vi "Output_file_Panel.vi"(8 "Show panel ?":bool, 9 "Channel Names":string[](array[string]), 10 "Header":string, 11 "Output filename":path=path "/G3_3 HD/Users/Paul/New Disp DB file") -> (0 "Save Full Res Data?":bool, 1 "Desired Columns":i32[](array[numeric]), 2 "Header Out":string, 3 "Output filename Out":path=path "/G3_3 HD/Users/Paul/New Disp DB file", 4 "Channels to Tabulate in header Out":i32[](listbox), 5 "Save Plotted rows only?":bool, 6 "Summarise mode":T1(ring), 7 "Grouping info":T3[](array[typedef]))   [LabVIEW 2016]
uses:
  Controls/Group_Binning.ctl
  Results_plotter_Global.vi
panel:
  out "Raw data file index":i32
  in  "Channels to Tabulate in header":i32[](listbox)
  in  "Channels to first \"bin\" then output":i32[](listbox)
  in  "Channels to Ouput":i32[](listbox)
  in  "Channel to bin":T2(array[cluster])
  in  "Summarize data":i32(listbox)=2
  in  "OK Button":bool
  in  "Column Selector":i32(listbox)
  in  "Row Selector":i32(listbox)=1
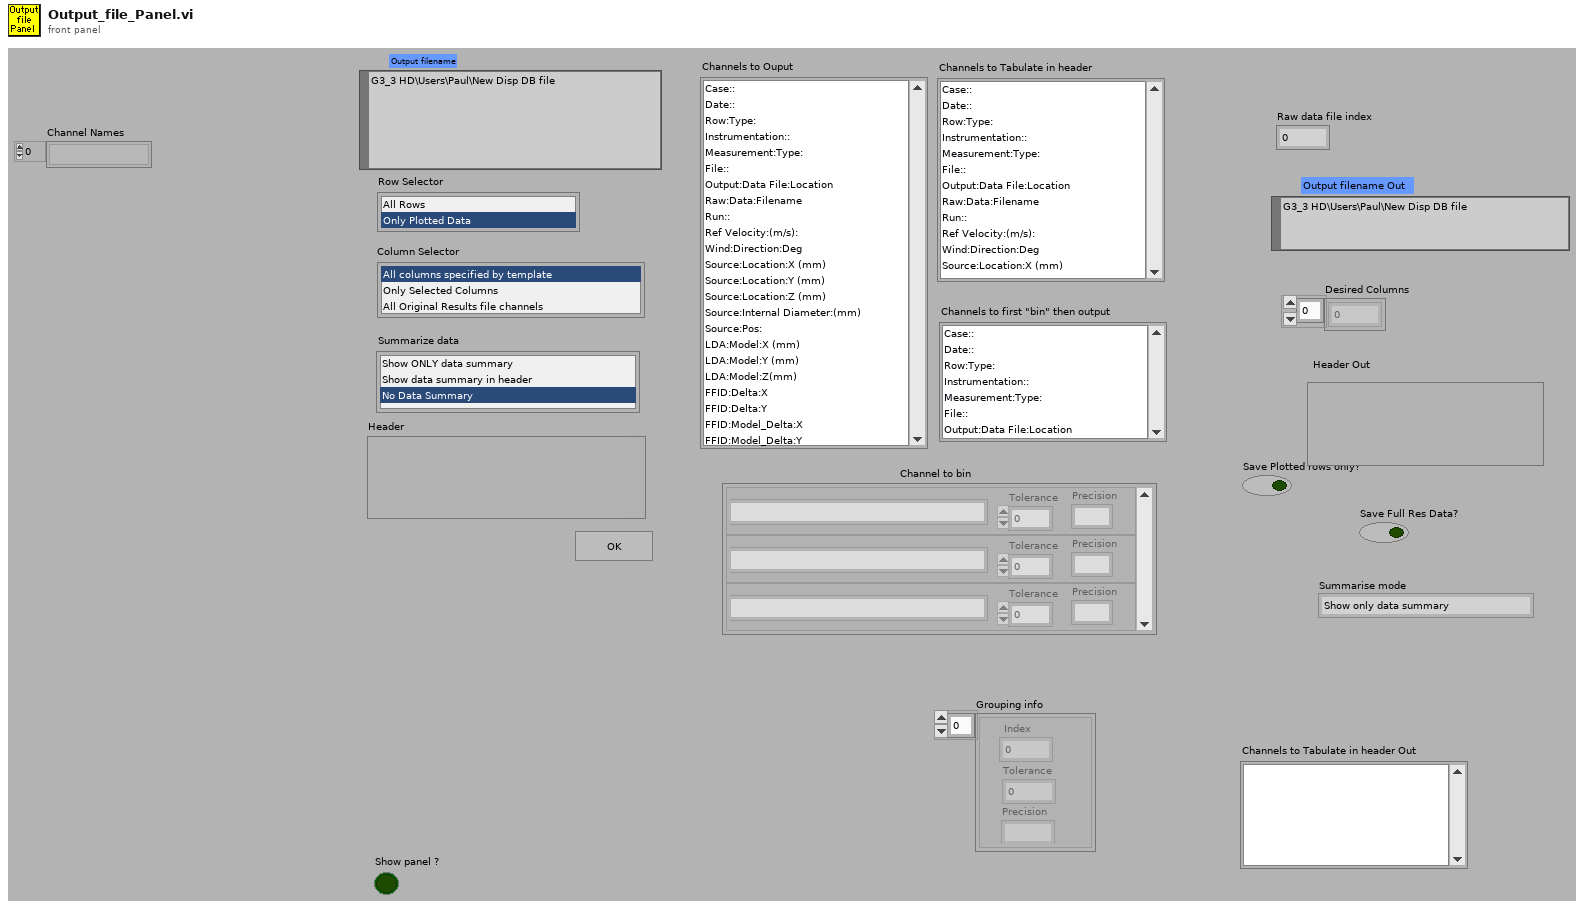
[diagram p1: front panel]
types:
  T1 = enum16{"Show only data summary", "Show data summary", "No data summary"}
  T2 = cluster{"Ch Name":string, "Tolerance":dbl, "Precision":string}[]
  T3 = typedef "Group_Binning.ctl" = cluster{"Index":i32, "Tolerance":dbl, "Precision":string}
  T4 = typedef "Dispose_Channel.ctl" = enum16{"Always", "If Blank", "Never"}
  T5 = cluster{"Ch Name":string, "Tolerance":dbl, "Precision":string}
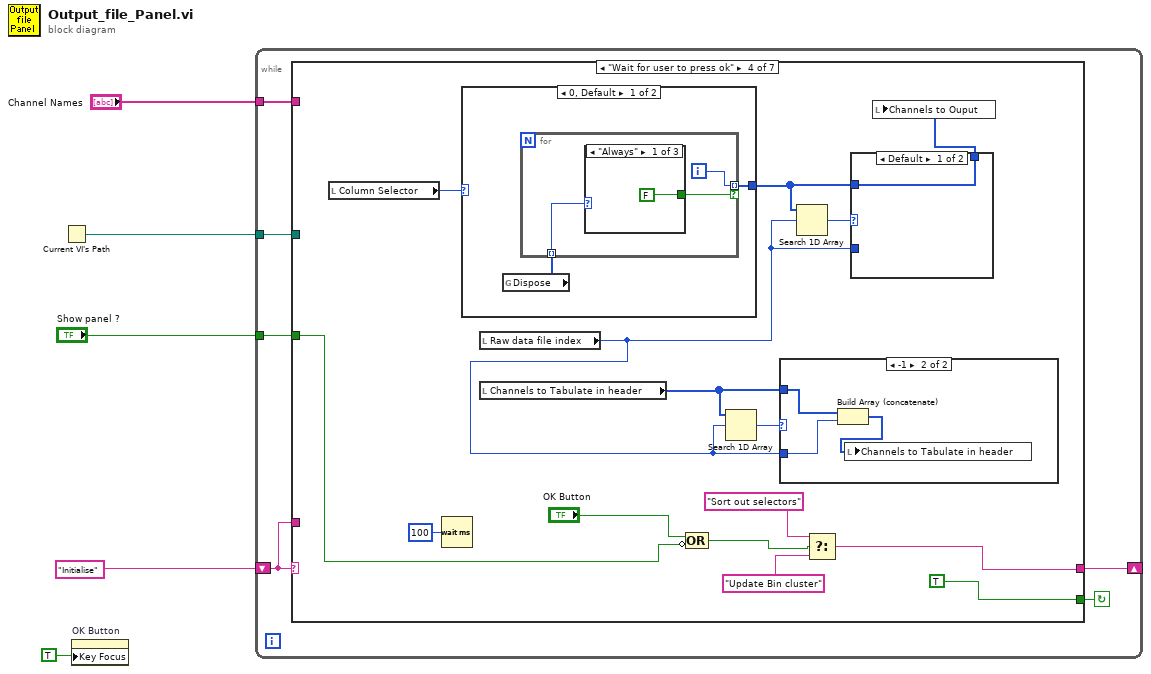
[diagram p0: block diagram]
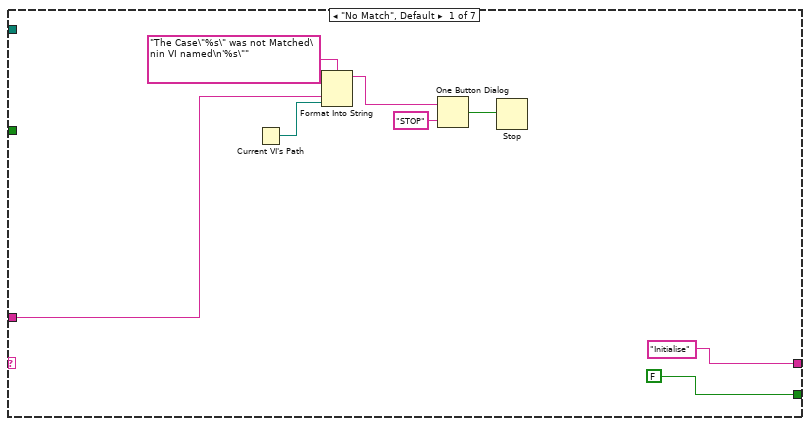
[diagram p2: hidden frame]
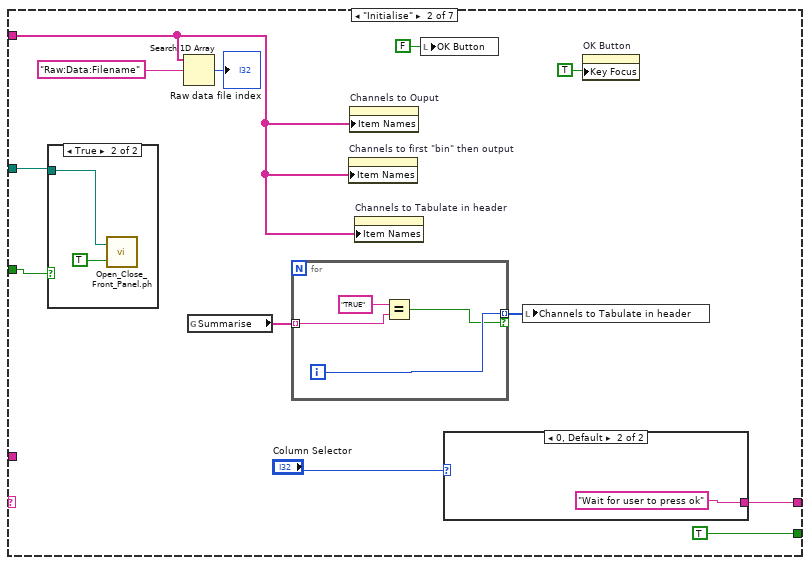
[diagram p3: hidden frame]
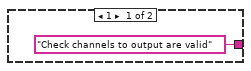
[diagram p4: hidden frame]
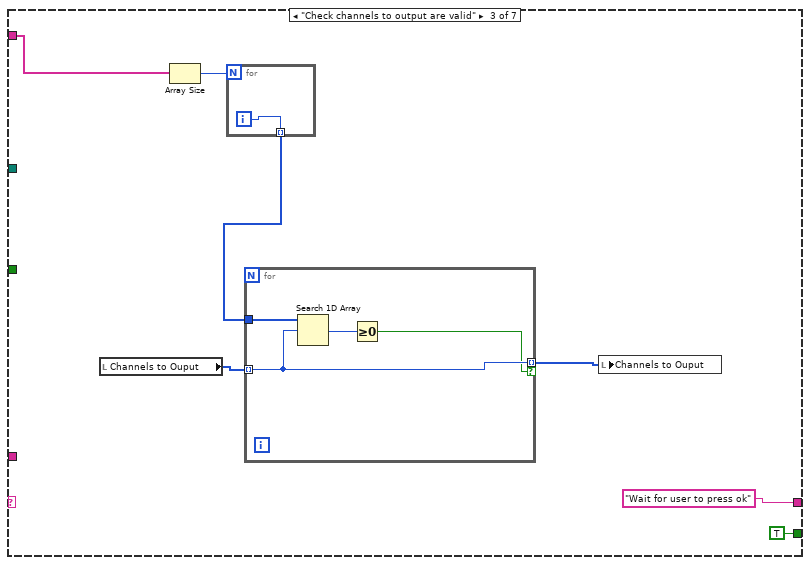
[diagram p6: hidden frame]
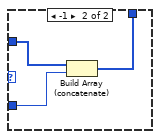
[diagram p8: hidden frame]
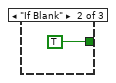
[diagram p9: hidden frame]
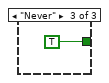
[diagram p10: hidden frame]
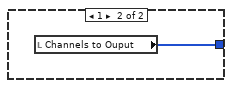
[diagram p11: hidden frame]
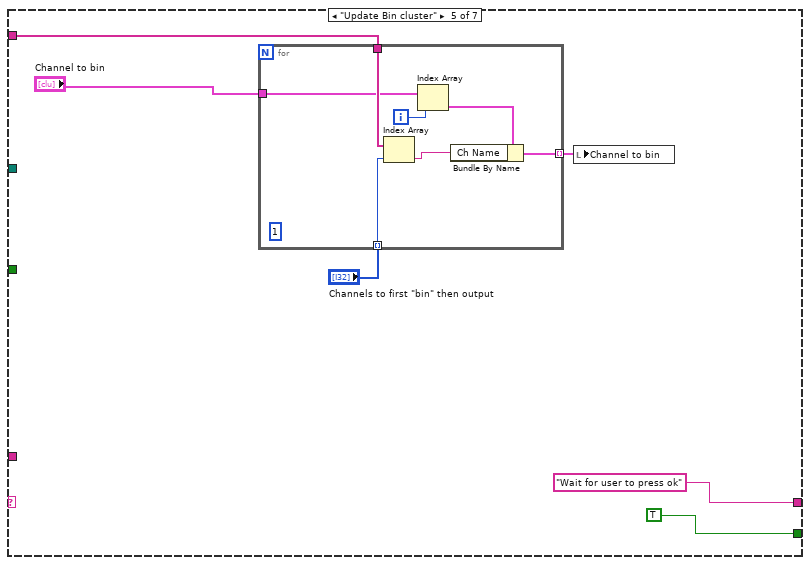
[diagram p12: hidden frame]
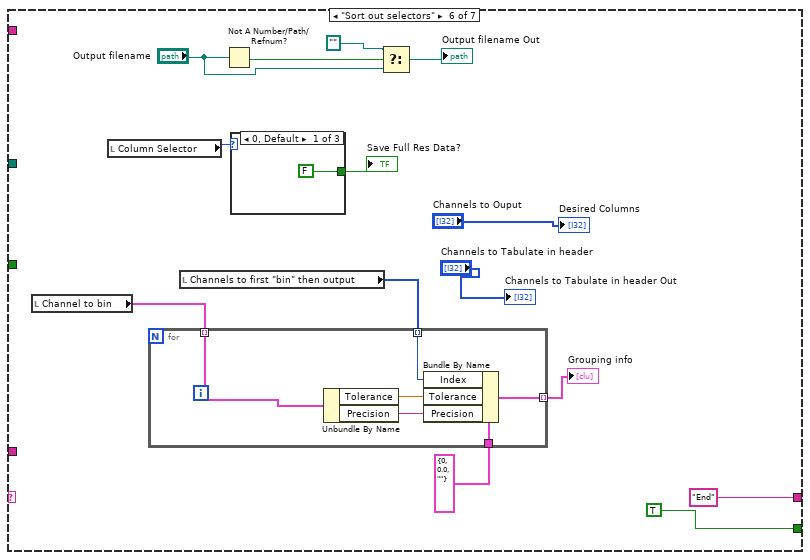
[diagram p13: hidden frame]
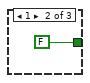
[diagram p14: hidden frame]
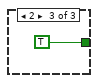
[diagram p15: hidden frame]
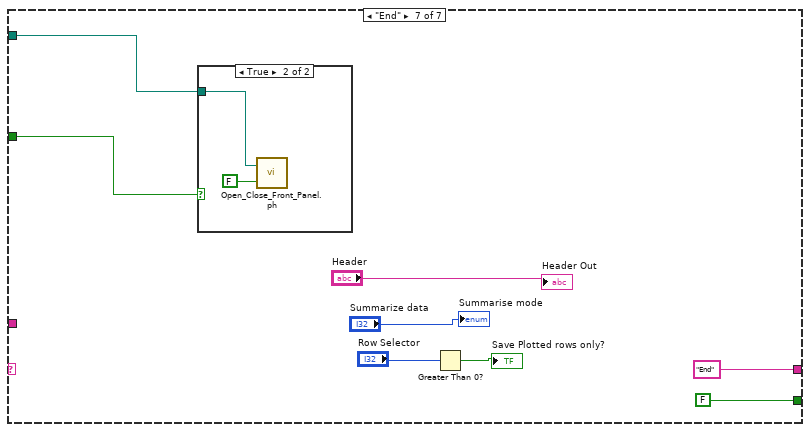
[diagram p16: hidden frame]
diagram:
  n1 = Current VI's Path() -> (path=w3:path)
  n2 = property on="OK Button" class="Bool (strict)"("Key Focus"=TRUE) -> ()  [unwired: 2 in, 2 out]
  n3 = while {
    shift-left: "Initialise" -> [w9]
    shift-right: [w10] -> _
    tunnel: "Show panel ?" -> [w8]
    tunnel: w3 -> [w7]
    tunnel: "Channel Names" -> [w6]
    stop <- w11 continue-if-true
    n4 = case shown="\"Wait for user to press ok\"" w9 {
      tunnel: [FALSE TRUE TRUE TRUE TRUE TRUE FALSE] -> w11
      tunnel: ["Initialise" w31 "Wait for user to press ok" w65 "Wait for user to press ok" "End" ("t") "End"] -> w10
      tunnel: w9 -> [w14 _ _ _ _ _ _]
      tunnel: w8 -> [_ w28 _ w59 _ _ w124]
      tunnel: w7 -> [_ w29 _ _ _ _ w123]
      tunnel: w6 -> [_ w21 w45 _ w85 _ _]
      frame "No Match", Default {
        n5 = Current VI's Path() -> (path=w13:path)
        n6 = Format Into String(format string="The Case\"%s\" was not Matched\nin VI named\n'%s\"" ("Format String"), w14, w13) -> (resulting string=w17:string)  [unwired: 2 in, 1 out]
        n7 = One Button Dialog(message=w17, button name ("OK")="STOP") -> (true=w15:bool)
        n8 = Stop(stop? (T)=w15) -> ()
      }
      frame "Initialise" {
        n9 = case shown="True" w28 {
          tunnel: w29 -> [_ w35]
          frame False {
          }
          frame True {
            n10 = call "Open_Close_Front_Panel.ph.vi"("Front Panel Window:Open"=TRUE, "VI path"=w35) -> ()  [unwired: 2 out]
          }
        }
        n11 = Search 1D Array(1D array=w21, element="Raw:Data:Filename" ("y")) -> (index of element=→"Raw data file index":i32)  [unwired: 1 in]
        n12 = global read "Results_plotter_Global.vi" "Summarise"() -> (w25:string[])
        n13 = for {
          tunnel: w25 -> [w38] mode=indexing
          tunnel: [w37] -> w24 mode=indexing if=w36
          i -> [w37]
          n14 = Equal?(x="TRUE", y=w38) -> (x = y?=w36:bool)
        }
        n15 = property on="Channels to first \"bin\" then output" class="LstBox (strict)"("Item Names"=w21) -> ()  [unwired: 2 in, 2 out]
        n16 = property on="Channels to Ouput" class="LstBox (strict)"("Item Names"=w21) -> ()  [unwired: 2 in, 2 out]
        n17 = property on="Channels to Tabulate in header" class="LstBox (strict)"("Item Names"=w21) -> ()  [unwired: 2 in, 2 out]
        n18 = local write "OK Button"(FALSE ("OK Button")) -> ()
        n19 = case shown="0, Default" "Column Selector" {
          tunnel: ["Check channels to output are valid" "Wait for user to press ok"] -> w31
          frame 1 {
          }
          frame 0, Default {
          }
        }
        n20 = local write "Channels to Tabulate in header"(w24) -> ()
        n21 = property on="OK Button" class="Bool (strict)"("Key Focus"=TRUE) -> ()  [unwired: 2 in, 2 out]
      }
      frame "Check channels to output are valid" {
        n22 = local read "Channels to Ouput"() -> (w44:i32[])
        n23 = Array Size(array=w45) -> (size(s)=w46:i32)
        n24 = for {
          N: w46 -> [_]
          tunnel: [w51] -> w43 mode=indexing
          i -> [w51]
        }
        n25 = for {
          tunnel: w44 -> [w49] mode=indexing
          tunnel: w43 -> [w50]
          tunnel: [w49] -> w42 mode=indexing if=w47
          n26 = Search 1D Array(1D array=w50, element=w49) -> (index of element=w48:i32)  [unwired: 1 in]
          n27 = Greater Or Equal To 0?(x=w48) -> (x >= 0?=w47:bool)
        }
        n28 = local write "Channels to Ouput"(w42) -> ()
      }
      frame "Wait for user to press ok" {
        n29 = local read "Column Selector"() -> (w52:i32)
        n30 = Wait (ms)(milliseconds to wait=u32 100) -> ()  [unwired: 1 out]
        n31 = case shown="0, Default" w52 {
          tunnel: [w74 w82] -> w57
          frame 0, Default {
            n32 = global read "Results_plotter_Global.vi" "Dispose"() -> (w75:T4[])
            n33 = for {
              tunnel: w75 -> [w78] mode=indexing
              tunnel: [w77] -> w74 mode=indexing if=w76
              i -> [w77]
              n34 = case shown="\"Always\"" w78 {
                tunnel: [FALSE TRUE TRUE] -> w76
                frame "Always" {
                }
                frame "If Blank" {
                }
                frame "Never" {
                }
              }
            }
          }
          frame 1 {
            n35 = local read "Channels to Ouput"() -> (w82:i32[])
          }
        }
        n36 = local read "Raw data file index"() -> (w53:i32)
        n37 = local read "Channels to Tabulate in header"() -> (w54:i32[])
        n38 = Compound Arithmetic op=OR("OK Button", invert w59) -> (w60:bool)
        n39 = Search 1D Array(1D array=w54, element=w53) -> (index of element=w55:i32)  [unwired: 1 in]
        n40 = case shown="-1" w55 {
          tunnel: w54 -> [_ w69]
          tunnel: w53 -> [_ w68]
          frame Default {
          }
          frame -1 {
            n41 = Build Array (concatenate)(w69, w68) -> (w67:i32[])
            n42 = local write "Channels to Tabulate in header"(w67) -> ()
          }
        }
        n43 = Search 1D Array(1D array=w57, element=w53) -> (index of element=w58:i32)  [unwired: 1 in]
        n44 = Select(t="Sort out selectors", s=w60, f="Update Bin cluster") -> (s? t:f=w65:string)
        n45 = case shown="Default" w58 {
          tunnel: w57 -> [w70 w73]
          tunnel: w53 -> [_ w72]
          tunnel: [w70 w71] -> w56
          frame Default {
          }
          frame -1 {
            n46 = Build Array (concatenate)(w73, w72) -> (w71:i32[])
          }
        }
        n47 = local write "Channels to Ouput"(w56) -> ()
      }
      frame "Update Bin cluster" {
        n48 = for {
          tunnel: "Channels to first \"bin\" then output" -> [w95] mode=indexing
          tunnel: w85 -> [w94]
          tunnel: "Channel to bin" -> [w91]
          tunnel: [w89] -> w83 mode=indexing
          i -> [w92]
          (unwired) 1 ("length (rest)")
          n49 = Index Array(array=w94, index=w95) -> (element=w93:string)
          n50 = Index Array(array=w91, index=w92) -> (element=w90:T5)
          n51 = Bundle By Name(cluster=w90, "Ch Name"=w93) -> (w89:T5)
        }
        n52 = local write "Channel to bin"(w83) -> ()
      }
      frame "Sort out selectors" {
        n53 = local read "Channel to bin"() -> (w101:T2)
        n54 = local read "Column Selector"() -> (w108:i32)
        n55 = local read "Channels to first \"bin\" then output"() -> (w98:i32[])
        n56 = for {
          tunnel: w101 -> [w115] mode=indexing
          tunnel: [w112] -> w100 mode=indexing
          tunnel: w98 -> [w111] mode=indexing
          tunnel: T3 {"Index"=0, "Tolerance"=0.0, "Precision"=""} ("Grouping info") -> [w110]
          n57 = Unbundle By Name(w115) -> ("Tolerance"=w114:dbl, "Precision"=w113:string)
          n58 = Bundle By Name(cluster=w110, "Index"=w111, "Tolerance"=w114, "Precision"=w113) -> (w112:T3)
        }
        "Grouping info" <- w100
        n59 = Not A Number/Path/Refnum?(number/path/refnum="Output filename") -> (NaN/Path/Refnum?=w105:bool)
        n60 = case shown="0, Default" w108 {
          tunnel: [FALSE FALSE TRUE] -> w106
          frame 0, Default {
          }
          frame 1 {
          }
          frame 2 {
          }
        }
        "Save Full Res Data?" <- w106
        n61 = Select(t=path "", s=w105, f="Output filename") -> (s? t:f=→"Output filename Out":path)
        "Desired Columns" <- "Channels to Ouput"
        "Channels to Tabulate in header Out" <- "Channels to Tabulate in header"
      }
      frame "End" {
        n62 = case shown="True" w124 {
          tunnel: w123 -> [_ w128]
          frame False {
          }
          frame True {
            n63 = call "Open_Close_Front_Panel.ph.vi"("Front Panel Window:Open"=FALSE, "VI path"=w128) -> ()  [unwired: 2 out]
          }
        }
        n64 = Greater Than 0?(x="Row Selector") -> (x > 0?=→"Save Plotted rows only?":bool)
        "Header Out" <- "Header"
        "Summarise mode" <- "Summarize data"
      }
    }
  }
